vi "q1 histiograph histiogram.vi"() -> ()   [LabVIEW 2018]
uses:
  <vilib>/vision/NI_Vision_Development_Module.lvlib
panel:
  out "Histogram Report":T1 {"Standard  Variation" format="%.2f"; "Mean Value" format="%.2f"; "Interval Width" format="%.2f"; "Starting Value" format="%.2f"; "Maximal Value" format="%.2f"; "Minimal Value" format="%.2f"}
  out "Waveform Graph":T2(graph)
  in  "Use File Path Image Type":bool=TRUE
  out "Image":T3(plugin-control)
  in  "File Path":path
  in  "Image Type":T4 items=["Grayscale (U8)", "Grayscale (I16)", "Grayscale (SGL)", "Complex (CSG)", "RGB (U32)", "HSL (U32)", "RGB (U64)", "Grayscale (U16)"]
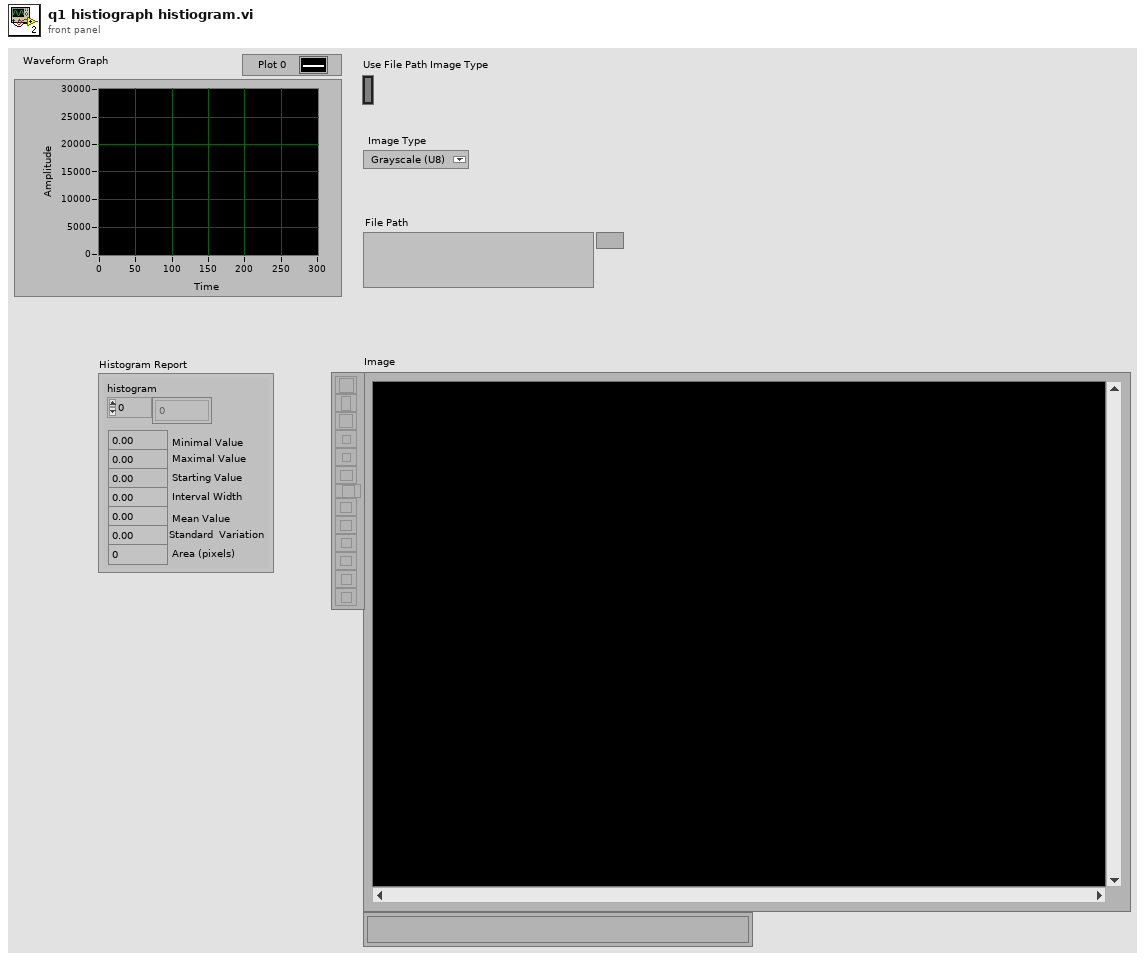
[diagram p1: front panel]
types:
  T1 = cluster{"histogram":u32[], "Minimal Value":sgl, "Maximal Value":sgl, "Starting Value":sgl, "Interval Width":sgl, "Mean Value":sgl, "Standard  Variation":sgl, "Area (pixels)":i32}
  T2 = cluster{"Starting Value":sgl, "Incremental Value":sgl, "Histogram":u32[]}
  T3 = typedef "IMAQ Image.ctl" = refnum<image>
  T4 = typedef "Image Type" = u32
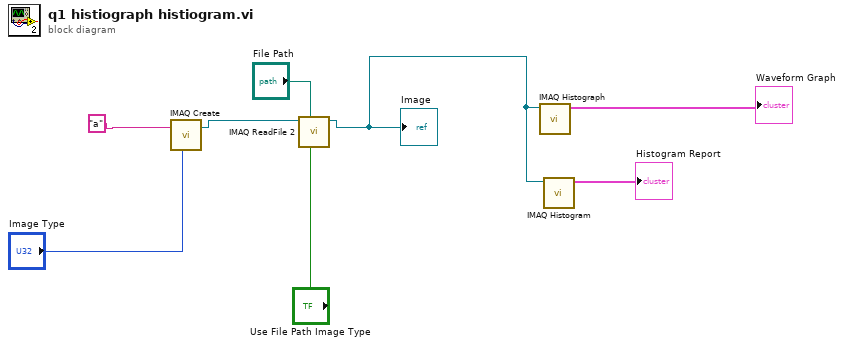
[diagram p0: block diagram]
diagram:
  n1 = call "IMAQ Create"("Image Name"="a", "Image Type"="Image Type") -> ("New Image"=w6:T3)  [unwired: 3 in, 1 out]
  n2 = call "IMAQ ReadFile 2"("Use File Path Image Type"="Use File Path Image Type", "File Path"="File Path", "Image"=w6) -> ("Image Out"=w2:T3)  [unwired: 4 in, 4 out]
  "Image" <- w2
  n3 = call "IMAQ Histograph"("Image"=w2) -> ("Histogram Graph"=→"Waveform Graph":T2)  [unwired: 7 in, 3 out]
  n4 = call "IMAQ Histogram"("Image"=w2) -> ("Histogram Report"=→"Histogram Report":T1)  [unwired: 9 in, 1 out]
